vi "NanonisFrame1.vi"(2 "Nano Z Write (m)":dbl, 3 "Begin Writing?":bool, 6 "x (nm)":dbl, 8 "z (nm)":dbl) -> (12 "Speed (nm/s)":dbl, 15 "Frame Parameters (m)":T1, 16 "Setpoint Current (A)":dbl, 17 "Current (A)":dbl, 19 "Nano Z Read (m)":sgl format="%#_6p")   [LabVIEW 2019]
uses:
  <instrlib>/Nanonis Prog Interface V5/Nanonis Prog Interface.lvlib
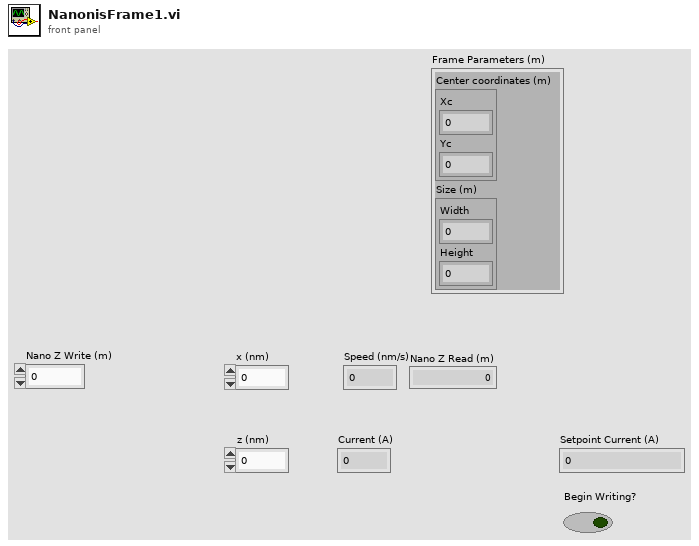
[diagram p1: front panel]
types:
  T1 = cluster{"Center coordinates (m)":cluster{"Xc":sgl, "Yc":sgl}, "Size (m)":cluster{"Width":sgl, "Height":sgl}}
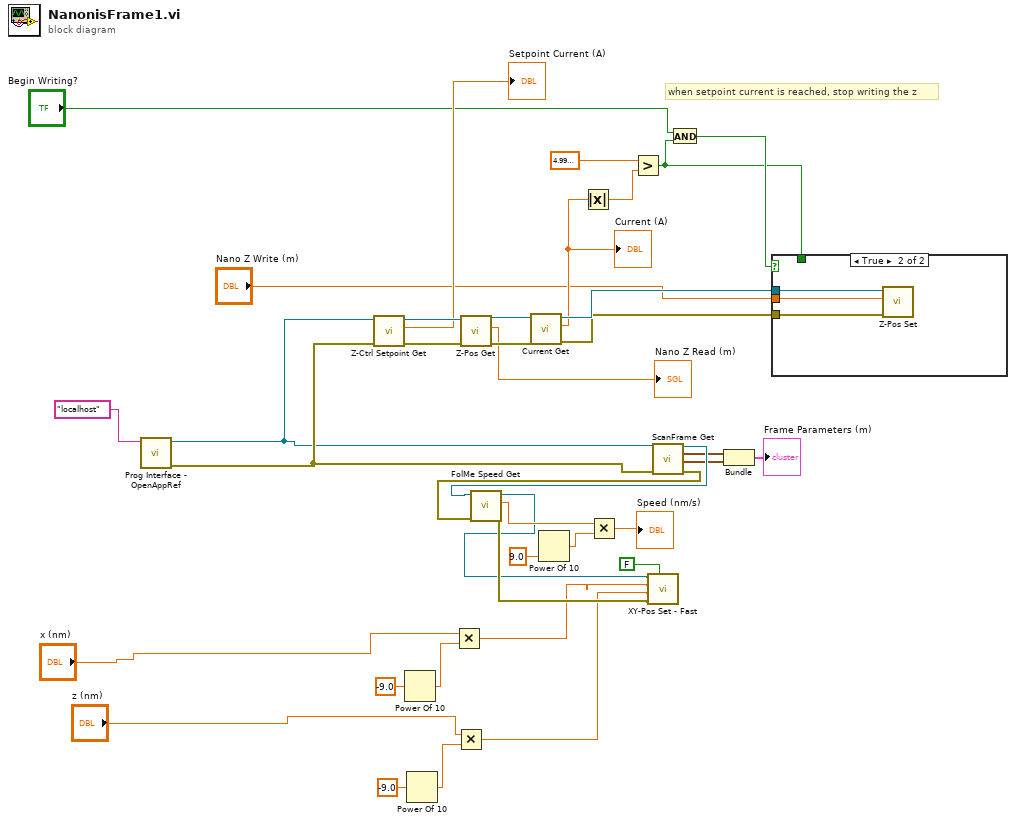
[diagram p0: block diagram]
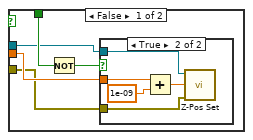
[diagram p2: hidden frame]
diagram:
  # "when setpoint current is reached, stop writing the z"
  n1 = call <instrlib>:"Prog Interface - OpenAppRef.vi"("Machine name (local machine IP)"="localhost") -> ("Error out"=w16:errorcluster, "Application reference"=w15:refnum<vi>)  [unwired: 5 in]
  n2 = call <instrlib>:"Z-Ctrl Setpoint Get.vi"("error in (no error)"=w16, "Application ref in"=w15) -> ("error out"=w17:errorcluster, "Z Controller setpoint"=→"Setpoint Current (A)":sgl, "Application ref out"=w18:refnum<vi>)  [unwired: 6 in]
  n3 = Power Of 10(x=-9.0) -> (10^x=w32:dbl)
  n4 = Power Of 10(x=-9.0) -> (10^x=w30:dbl)
  n5 = Multiply(x="x (nm)", y=w32) -> (x*y=w23:dbl)
  n6 = Multiply(x="z (nm)", y=w30) -> (x*y=w24:dbl)
  n7 = call <instrlib>:"Z-Pos Get.vi"("error in (no error)"=w17, "Application ref in"=w18) -> ("error out"=w19:errorcluster, "Z position (m)"=→"Nano Z Read (m)":sgl, "Application ref out"=w20:refnum<vi>)  [unwired: 7 in]
  n8 = call <instrlib>:"Current Get.vi"("Error in (no error)"=w19, "Application ref in"=w20) -> ("Error out"=w13:errorcluster, "Current (A)"=w11:sgl, "Application ref out"=w14:refnum<vi>)  [unwired: 5 in]
  "Current (A)" <- w11
  n9 = Power Of 10(x=9.0) -> (10^x=w35:dbl)
  n10 = Absolute Value(x=w11) -> (abs(x)=w12:sgl)
  n11 = Greater?(x=sgl 5e-09, y=w12) -> (0:w7:bool)
  n12 = call <instrlib>:"ScanFrame Get.vi"("Application ref in"=w15, "error in (no error)"=w16) -> ("Application ref out"=w37:refnum<vi>, "Center coordinates (m)"=w5:cluster{"Xc":sgl, "Yc":sgl}, "Size (m)"=w4:cluster{"Width":sgl, "Height":sgl}, "error out"=w28:errorcluster)  [unwired: 9 in, 1 out]
  n13 = call <instrlib>:"FolMe Speed Get.vi"("error in (no error)"=w28, "Application ref in"=w37) -> ("error out"=w25:errorcluster, "Speed (m/s)"=w34:sgl, "Application ref out"=w22:refnum<vi>)  [unwired: 4 in, 1 out]
  n14 = Multiply(x=w34, y=w35) -> (x*y=→"Speed (nm/s)":dbl)
  n15 = call <instrlib>:"XY-Pos Set - Fast.vi"("Wait end-of-motion (T=True)"=FALSE, "error in (no error)"=w25, "Y (m)"=w24, "X (m)"=w23, "Application ref in"=w22) -> ()  [unwired: 4 in, 2 out]
  n16 = And(x="Begin Writing?", y=w7) -> (x .and. y?=w8:bool)
  n17 = Bundle("Center coordinates (m)"=w5, "Size (m)"=w4) -> (→"Frame Parameters (m)":T1)  [unwired: 1 in]
  n18 = case shown="True" w8 {
    tunnel: "Nano Z Write (m)" -> [w41 w51]
    tunnel: w14 -> [w40 w50]
    tunnel: w13 -> [w39 w49]
    tunnel: w7 -> [w43 _]
    frame False {
      n19 = Not(x=w43) -> (.not. x?=w42:bool)
      n20 = case shown="True" w42 {
        tunnel: w41 -> [_ w47]
        tunnel: w40 -> [_ w45]
        tunnel: w39 -> [_ w44]
        frame False {
        }
        frame True {
          n21 = Add(x=w47, y=1e-09) -> (x+y=w48:dbl)
          n22 = call <instrlib>:"Z-Pos Set.vi"("error in (no error)"=w44, "Z position (m)"=w48, "Application ref in"=w45) -> ()  [unwired: 7 in, 2 out]
        }
      }
    }
    frame True {
      n23 = call <instrlib>:"Z-Pos Set.vi"("error in (no error)"=w49, "Z position (m)"=w51, "Application ref in"=w50) -> ()  [unwired: 7 in, 2 out]
    }
  }
